vi "Reynolds Number.vi"(6 "Effective Length (m)":dbl, 9 "Density (kg/m^3)":dbl, 10 "Viscosity (Pa-s)":dbl, 11 "Velocity (m/s)":dbl) -> (3 "Reynolds Number":dbl)   [LabVIEW 2019]
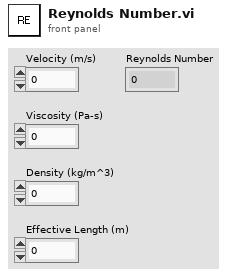
[diagram p1: front panel]
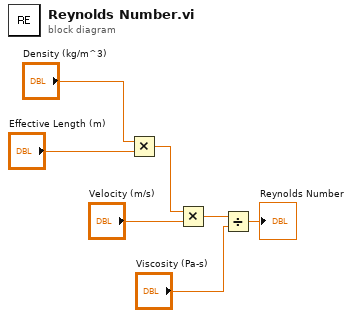
[diagram p0: block diagram]
diagram:
  n1 = Multiply(x="Density (kg/m^3)", y="Effective Length (m)") -> (x*y=w1:dbl)
  n2 = Multiply(x=w1, y="Velocity (m/s)") -> (x*y=w5:dbl)
  n3 = Divide(x=w5, y="Viscosity (Pa-s)") -> (x/y=→"Reynolds Number":dbl)
